vi "Init SM.vi"(7 "Event Queue":refnum<queue>, 11 "Work VI":refnum<vi>) -> (3 "Worker Block":T1={"Block Status"=refnum, "Command Queue"=refnum, "Status"={"Block Status"={"State"=enum."Init", "Next State"=enum."Idle", "Runs"=0, "i"=0, "Init"=FALSE, "Started"=FALSE, "Closing"=FALSE, "Step"=FALSE, "Phase"=enum."N/A", "Worker"=""}, "Error"={"status"=FALSE, "code"=0, "source"=""}}})   [LabVIEW 2022 SP3, in "FlexBlocks Support.lvlib"]
uses:
  FlexBlocks Support.lvlib
  Block State.ctl
  Block Phase.ctl
  Block Status.ctl
  Block Command.ctl
  Block Status with Error.ctl
  Worker Block.ctl
  Worker Registration.ctl
  Execution Events.ctl
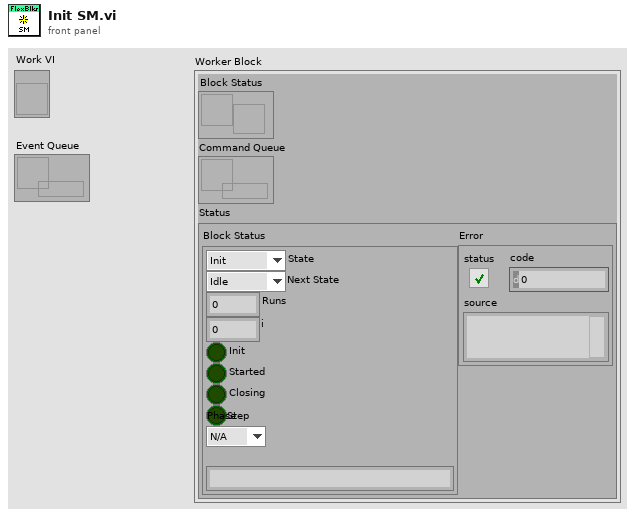
[diagram p1: front panel]
types:
  T1 = typedef "FlexBlocks Support.lvlib/Worker Block.ctl" = cluster{"Block Status":refnum<user-event>, "Command Queue":refnum<queue>, "Status":T2}
  T2 = typedef "FlexBlocks Support.lvlib/Block Status with Error.ctl" = cluster{"Block Status":T3, "Error":errorcluster}
  T3 = typedef "FlexBlocks Support.lvlib/Block Status.ctl" = cluster{"State":T4, "Next State":T4, "Runs":u32, "i":i32, "Init":bool, "Started":bool, "Closing":bool, "Step":bool, "Phase":T5, "Worker":string}
  T4 = typedef "FlexBlocks Support.lvlib/Block State.ctl" = enum16{"Idle", "Init", "Start", "Run", "Stop", "Close"}
  T5 = typedef "FlexBlocks Support.lvlib/Block Phase.ctl" = enum16{"N/A", "Read", "Work", "Write"}
  T6 = typedef "FlexBlocks Support.lvlib/Worker Registration.ctl" = cluster{"Worker":string, "Response":refnum<notifier>}
  T7 = typedef "FlexBlocks Support.lvlib/Execution Events.ctl" = cluster{"Registration":refnum<user-event>, "Init":refnum<user-event>, "Run":refnum<user-event>, "Step":refnum<user-event>, "Stop":refnum<user-event>, "Close":refnum<user-event>, "Block Status":refnum<user-event>}
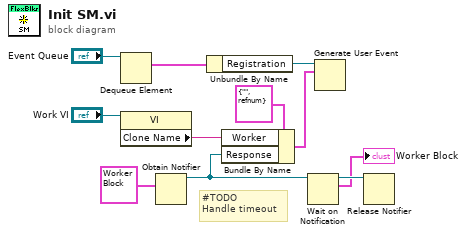
[diagram p0: block diagram]
diagram:
  # "#TODO\nHandle timeout"
  n1 = Dequeue Element(queue="Event Queue") -> (element=w1:T7)  [unwired: 2 in, 3 out]
  n2 = property class="VI"(reference="Work VI") -> ("Clone Name"=w7:string)  [unwired: 1 in, 2 out]
  n3 = Obtain Notifier(notification data type=T1 {"Block Status"=refnum, "Command Queue"=refnum, "Status"={"Block Status"={"State"=enum."Init", "Next State"=enum."Idle", "Runs"=0, "i"=0, "Init"=FALSE, "Started"=FALSE, "Closing"=FALSE, "Step"=FALSE, "Phase"=enum."N/A", "Worker"=""}, "Error"={"status"=FALSE, "code"=0, "source"=""}}} ("Worker Block")) -> (notifier out=w6:refnum<notifier>)  [unwired: 3 in, 2 out]
  n4 = Unbundle By Name(w1) -> ("Registration"=w3:refnum<user-event>)
  n5 = Bundle By Name(cluster=T6 {"Worker"="", "Response"=refnum} ("event data"), "Worker"=w7, "Response"=w6) -> (w8:T6)
  n6 = Wait on Notification(notifier=w6) -> (notifier out=w5:refnum<notifier>, notification=→"Worker Block":T1)  [unwired: 3 in, 2 out]
  n7 = Generate User Event(user event=w3, event data cluster=w8) -> ()  [unwired: 2 in, 2 out]
  n8 = Release Notifier(notifier=w5) -> ()  [unwired: 2 in, 3 out]
